vi "v1h_get_NC_attr.vi"(3 "errorin":errorcluster caption="error in", 5 "refnum in":refnum<file>) -> (0 "error out":errorcluster, 1 "NC_attr":T1 {"nc_type" items=["NC_NAT", "NC_BYTE", "NC_CHAR", "NC_SHORT", "NC_INT", "NC_FLOAT", "NC_DOUBLE"]}, 2 "refnum out":refnum<file>)   [LabVIEW 2016]
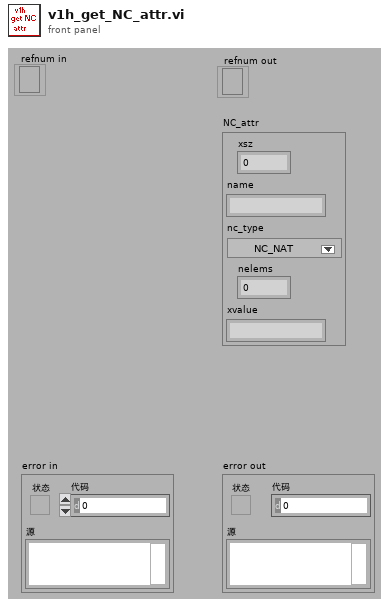
[diagram p1: front panel]
types:
  T1 = cluster{"xsz":u64, "name":string, "nc_type":u16, "nelems":u64, "xvalue":string}
  T2 = enum16{"big-endian, network order", "native, host order", "little-endian"}
  T3 = cluster{"size":i32, "NC_string":string, "int32":i32, "int32":i32, string}
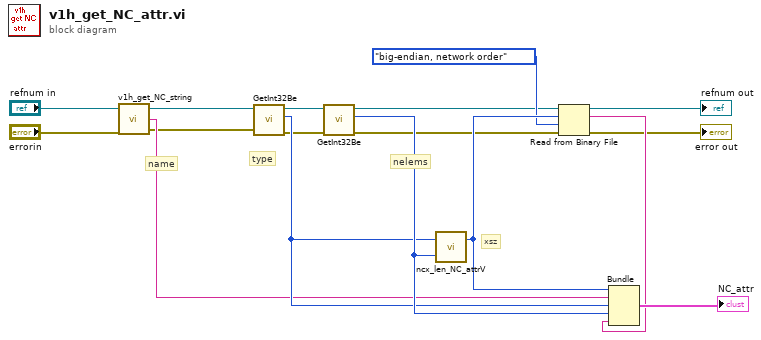
[diagram p0: block diagram]
diagram:
  # "xsz"
  # "name"
  # "nelems"
  # "type"
  n1 = call "v1h_get_NC_string.vi"("error in (no error)"="errorin", "refnum in"="refnum in") -> ("error out"=w1:errorcluster, "NC_string"=w15:string, "refnum out"=w4:refnum<file>)  [unwired: 1 out]
  n2 = call "GetInt32Be.vi"("error in (no error)"=w1, "refnum in"=w4) -> ("error out"=w9:errorcluster, "int32"=w16:i32, "refnum out"=w5:refnum<file>)  [unwired: 3 out]
  n3 = call "GetInt32Be.vi"("error in (no error)"=w9, "refnum in"=w5) -> ("error out"=w10:errorcluster, "int32"=w17:i32, "refnum out"=w7:refnum<file>)  [unwired: 3 out]
  n4 = call "ncx_len_NC_attrV.vi"("nelems"=w17, "nc_type"=w16) -> ("size"=w13:i32)  [unwired: 1 out]
  n5 = Read from Binary File(8:w10, 9:T2."big-endian, network order" ("字节顺序(0:big-endian, network order)"), 10:w13, 11:w7) -> (0:→"error out":errorcluster, 2:w12:string, 3:→"refnum out":refnum<file>)  [unwired: 3 out]
  n6 = Bundle("size"=w13, "NC_string"=w15, "int32"=w16, "int32"=w17, w12) -> (→"NC_attr":T3)  [unwired: 1 out]
